vi "Apply Filter_1D.vi"(10 "Filter":string, 11 "Item names":string[](array[string])) -> (3 "Filtered Item Names":string[](array[string]))   [LabVIEW 2013, in "CVT editor node.lvclass"]
uses:
  CVT editor node.lvclass
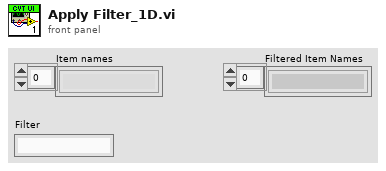
[diagram p1: front panel]
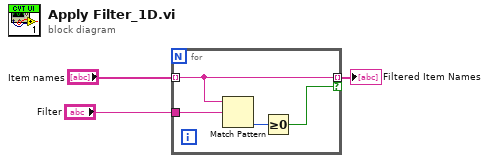
[diagram p0: block diagram]
diagram:
  n1 = for {
    tunnel: "Item names" -> [w6] mode=indexing
    tunnel: "Filter" -> [w7]
    tunnel: [w6] -> w1 mode=indexing if=w4
    n2 = Match Pattern(string=w6, regular expression=w7) -> (offset past match=w5:i32)  [unwired: 1 in, 3 out]
    n3 = Greater Or Equal To 0?(x=w5) -> (x >= 0?=w4:bool)
  }
  "Filtered Item Names" <- w1
